vi "CircularCenter.vi"(0 "controller in":refnum<k24>, 1 "axis 1 name":string, 2 "axis 1 endpoint":dbl, 3 "axis 2 name":string, 4 "axis 2 endpoint":dbl, 5 "error in (no error)":errorcluster, 6 "speed":dbl, 7 "axis 1 center point":dbl, 8 "direction":u16(ring) items=["Clockwise", "Counter-clockwise"], 9 "axis 2 center point":dbl, 11 "taskId":i32(ring) items=["TLibrary", "T01", "T02", "T03", "T04", "T05", "T06", "T07", "T08", "T09", "T10", "T11", "T12", "T13", "T14", "T15", "T16", "T17", "T18", "T19", "T20", "T21", "T22", "T23", "T24", "T25", "T26", "T27", "T28", "T29", "T30", "T31"], 13 "return immediately":bool) -> (14 "controller out":refnum<k24>, 19 "error out":errorcluster)   [LabVIEW 2019, in "Aerotech VIs.lvlib"]
uses:
  Aerotech VIs.lvlib
  C:/Program Files (x86)/Aerotech/A3200/LabVIEW/2010/Bin/Aerotech.A3200.dll
  Program Files (x86)/Aerotech/A3200/LabVIEW/2010/Bin/Aerotech.A3200.dll
  C:/Program Files (x86)/Aerotech/A3200/LabVIEW/2010/Bin/Aerotech.A3200.LabVIEW.dll
  Program Files (x86)/Aerotech/A3200/LabVIEW/2010/Bin/Aerotech.A3200.LabVIEW.dll
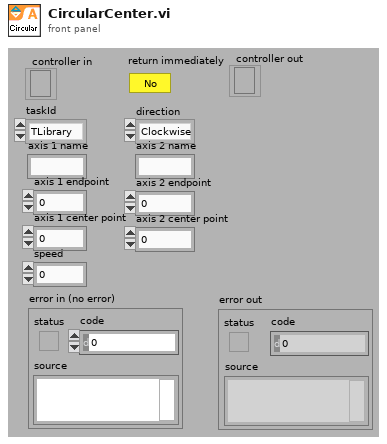
[diagram p1: front panel]
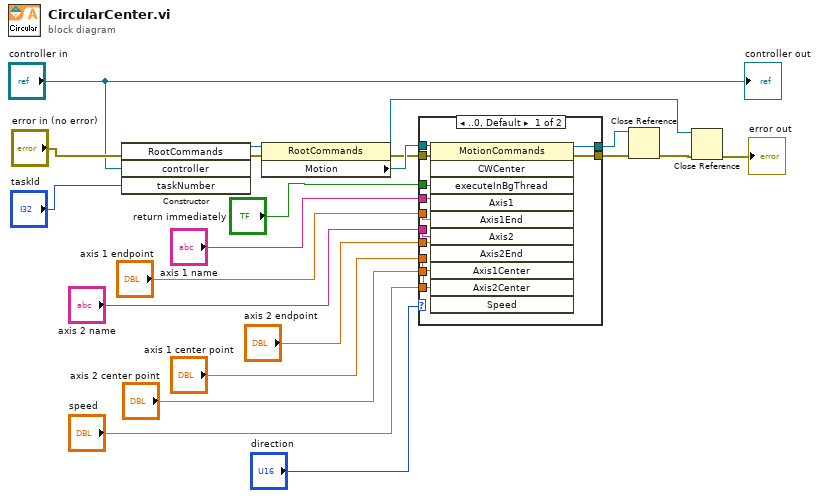
[diagram p0: block diagram]
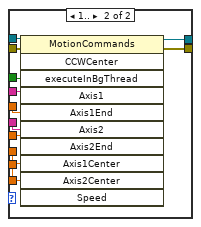
[diagram p2: hidden frame]
diagram:
  n1 = constructor class="RootCommands"(error in="error in (no error)", "controller"="controller in", "taskNumber"="taskId") -> (reference out=w7:refnum<k24>, error out=w6:errorcluster)  [unwired: 2 in, 3 out]
  n2 = property class="RootCommands"(reference=w7, error in=w6) -> (reference out=w2:refnum<k24>, error out=w8:errorcluster, "Motion"=w9:refnum<k24>)
  n3 = case shown="..0, Default" "direction" {
    tunnel: [w33 w43] -> w4
    tunnel: [w32 w42] -> w5
    tunnel: w8 -> [w31 w45]
    tunnel: w9 -> [w30 w44]
    tunnel: "speed" -> [w29 w34]
    tunnel: "axis 2 center point" -> [w28 w35]
    tunnel: "axis 1 center point" -> [w27 w36]
    tunnel: "axis 2 endpoint" -> [w26 w37]
    tunnel: "axis 2 name" -> [w25 w38]
    tunnel: "axis 1 endpoint" -> [w24 w39]
    tunnel: "axis 1 name" -> [w23 w40]
    tunnel: "return immediately" -> [w22 w41]
    frame ..0, Default {
      n4 = invoke class="MotionCommands" method="CWCenter"(reference=w30, error in=w31, "executeInBgThread"=w22, "Axis1"=w23, "Axis1End"=w24, "Axis2"=w25, "Axis2End"=w26, "Axis1Center"=w27, "Axis2Center"=w28, "Speed"=w29) -> (reference out=w33:refnum<k24>, error out=w32:errorcluster)  [unwired: 1 in, 9 out]
    }
    frame 1.. {
      n5 = invoke class="MotionCommands" method="CCWCenter"(reference=w44, error in=w45, "executeInBgThread"=w41, "Axis1"=w40, "Axis1End"=w39, "Axis2"=w38, "Axis2End"=w37, "Axis1Center"=w36, "Axis2Center"=w35, "Speed"=w34) -> (reference out=w43:refnum<k24>, error out=w42:errorcluster)  [unwired: 1 in, 9 out]
    }
  }
  n6 = Close Reference(reference=w4, error in (no error)=w5) -> (error out=w3:errorcluster)
  n7 = Close Reference(reference=w2, error in (no error)=w3) -> (error out=→"error out":errorcluster)
  "controller out" <- "controller in"
